vi "FTW-Supervisor-Core-Construct.vi"(0 "Initialization Sequence":string, 5 "FTW Supervisor Configuration":string, 11 "error in":errorcluster) -> (4 "FTW Supervisor":refnum<class "FTW-Supervisor.lvclass">, 6 "Incoming Request":refnum<event-registration>, 15 "error out":errorcluster)   [LabVIEW 2014, in "FTW-Supervisor.lvclass"]
uses:
  FTW-Supervisor.lvclass
  json/core/FTW-JSON-Core-Structure.ctl
  database/core/FTW-SQLite-Core-AccessMode.ctl
  FTW-Supervisor.lvclass/FTW-Supervisor.ctl
  lib/FTW-LibraryFilepath.vi
  reflection/FTW-Reflection-Type.vi
  error/FTW-ERR-ThrowGenericError.vi
  error/FTW-ERR-ThrowError.vi
  error/FTW-ERR-NoErrorConstant.vi
  json/FTW-JSON-Construct-FromBuffer.vi
  error/FTW-ERR-CallChain.vi
  string/FTW-STR-ReplaceWhitespace.vi
  reflection/FTW-Reflection-Array.vi
  json/core/FTW-JSON-Core-GetFlattenedValue.vi
  json/FTW-JSON-Destroy.vi
  json/FTW-JSON-Deserialize/FTW-JSON-Deserialize.xnode
  instance/FTW-Actor-Instance.lvclass
panel:
  # "Inputs"
  # "Outputs"
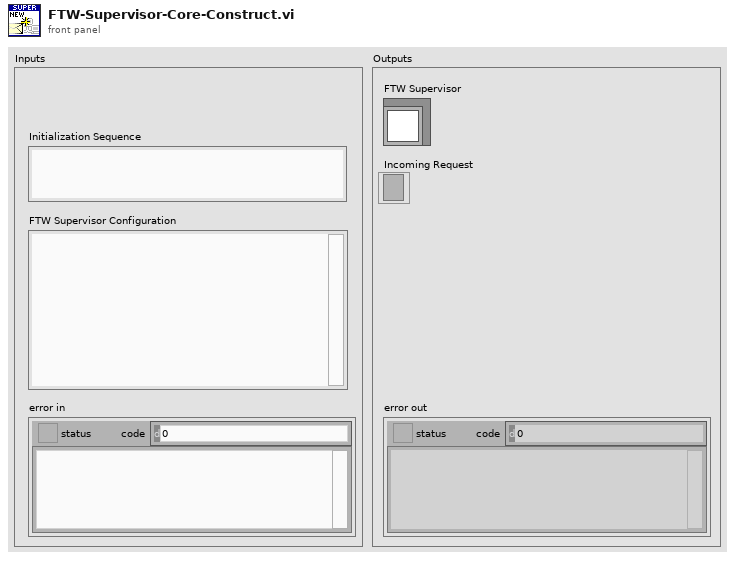
[diagram p1: front panel]
types:
  T1 = typedef "FTW-SQLite-Core-AccessMode.ctl" = enum16{"Read", "Read/Write", "Read/Write/Create"}
  T2 = cluster{"AppName":string, "AppVersionMajor":u32, "AppVersionMinor":u32, "AppVersionPatch":u32, "DashboardInboxAddress":string, "DashboardPublisherAddress":string, "DashboardPageAddress":string, "LogRetentionPolicy":cluster{"PersistToDisk":bool, "LogFilepath":path}}
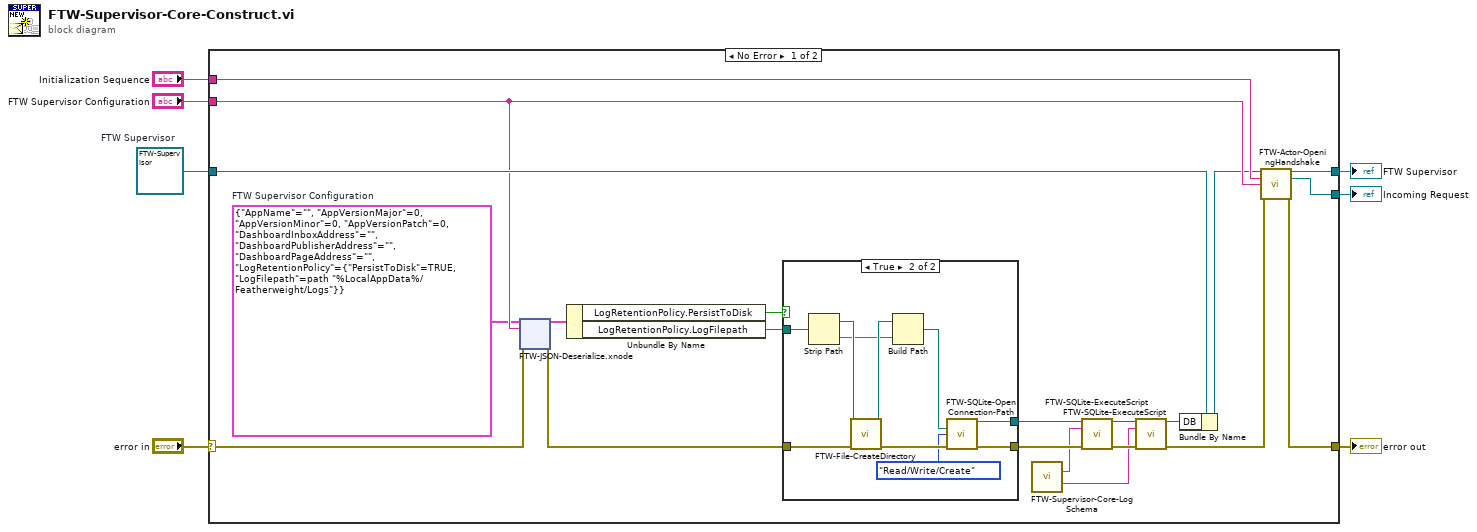
[diagram p0: block diagram]
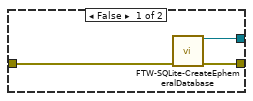
[diagram p2: hidden frame]
diagram:
  w7 = refnum<class "FTW-Supervisor.lvclass"> refnum  # FTW Supervisor
  n1 = case shown="No Error" "error in" {
    selector: "error in" -> [w23 w75]
    tunnel: [w26 w75] -> w5
    tunnel: [w28 w74] -> w1
    tunnel: w7 -> [w24 w74]
    tunnel: "FTW Supervisor Configuration" -> [w21 _]
    tunnel: [w27 _] -> w3
    tunnel: "Initialization Sequence" -> [w25 _]
    frame No Error {
      w20 = T2 {"AppName"="", "AppVersionMajor"=0, "AppVersionMinor"=0, "AppVersionPatch"=0, "DashboardInboxAddress"="", "DashboardPublisherAddress"="", "DashboardPageAddress"="", "LogRetentionPolicy"={"PersistToDisk"=TRUE, "LogFilepath"=path "%LocalAppData%/Featherweight/Logs"}}  # FTW Supervisor Configuration
      n2 = xnode "FTW-JSON-Deserialize.xnode"("Type and Defaults"=w20, "JSON String"=w21, "error in"=w23) -> ("Values"=w19:T2, "error out"=w22:errorcluster)  [unwired: 1 in]
      n3 = Unbundle By Name(w19) -> ("LogRetentionPolicy.PersistToDisk"=w17:bool, "LogRetentionPolicy.LogFilepath"=w18:path)
      n4 = case shown="True" w17 {
        tunnel: w22 -> [w29 w41]
        tunnel: [w31 w40] -> w15
        tunnel: [w30 w38] -> w14
        tunnel: w18 -> [_ w36]
        frame False {
          n5 = call "FTW-SQLite-CreateEphemeralDatabase.vi"("error in"=w29) -> ("SQLite Connection"=w31:refnum<data-value>, "error out"=w30:errorcluster)  [unwired: 13 in]
        }
        frame True {
          n6 = Strip Path(path=w36) -> (stripped path=w35:path, name=w32:string)
          n7 = call "FTW-File-CreateDirectory.vi"("Directory to Create"=w35, "error in"=w41) -> ("Created Directory"=w34:path, "error out"=w39:errorcluster)  [unwired: 12 in]
          n8 = Build Path(base path=w34, name or relative path=w32) -> (appended path=w33:path)
          n9 = call "FTW-SQLite-OpenConnection-Path.vi"("Database Filepath"=w33, "Access Mode"=FTW-SQLite-Core-AccessMode."Read/Write/Create", "error in"=w39) -> ("SQLite Connection"=w40:refnum<data-value>, "error out"=w38:errorcluster)  [unwired: 11 in]
        }
      }
      n10 = call "FTW-Supervisor-Core-LogSchema.vi"() -> ("Schema"=w13:string, "Indexes"=w8:string)  [unwired: 14 in]
      n11 = call "FTW-SQLite-ExecuteScript.vi"("SQLite Connection"=w15, "SQL Script"=w13, "error in"=w14) -> ("SQLite Connection out"=w9:refnum<data-value>, "error out"=w11:errorcluster)  [unwired: 10 in, 1 out]
      n12 = call "FTW-SQLite-ExecuteScript.vi"("SQLite Connection"=w9, "SQL Script"=w8, "error in"=w11) -> ("SQLite Connection out"=w12:refnum<data-value>, "error out"=w10:errorcluster)  [unwired: 10 in, 1 out]
      n13 = Bundle By Name(cluster=w24, "DB"=w12) -> (w16:refnum<class "FTW-Supervisor.lvclass">)
      n14 = call "FTW-Actor-OpeningHandshake.vi"("FTW Actor Instance Type"=w16, "Initialization Job Sequence"=w25, "Actor Instance Configuration"=w21, "error in"=w10) -> ("FTW Actor Instance"=w28:refnum<class "FTW-Supervisor.lvclass">, "Incoming Request"=w27:refnum<event-registration>, "error out"=w26:errorcluster)  [unwired: 9 in]
    }
    frame Error {
    }
  }
  "error out" <- w5
  "FTW Supervisor" <- w1
  "Incoming Request" <- w3
